vi "Set Exposure Time.vi"(8 "error in (no error)":errorcluster, 10 "Exposure Time (s)":dbl, 11 "Abstract Camera in":refnum<class "Abstract Camera.lvclass">) -> (0 "error out":errorcluster, 2 "Exposure Time (s) out":dbl, 3 "Abstract Camera out":refnum<class "Abstract Camera.lvclass">)   [LabVIEW 2019, in "Abstract Camera.lvclass"]
uses:
  Abstract Camera.lvclass
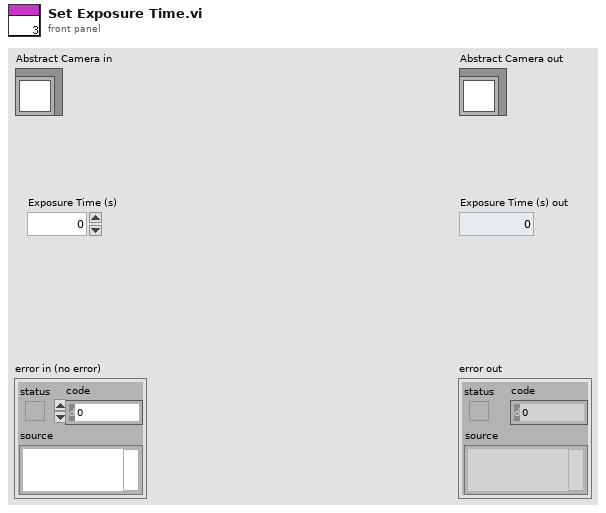
[diagram p1: front panel]
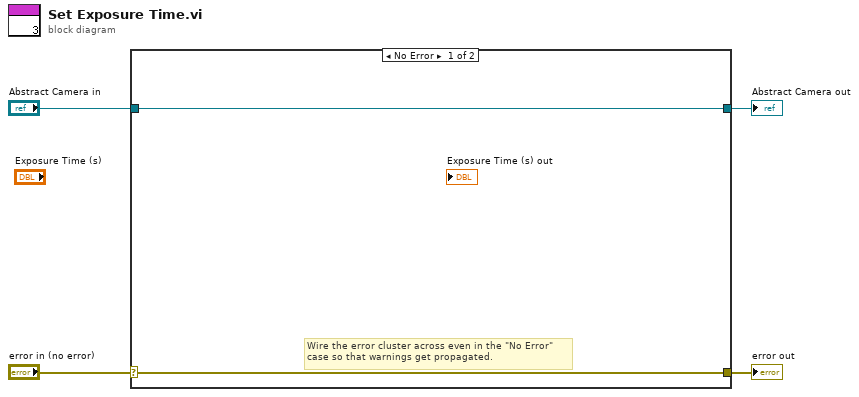
[diagram p0: block diagram]
diagram:
  n1 = case shown="No Error" "error in (no error)" {
    selector: "error in (no error)" -> [w5 w8]
    tunnel: [w5 w8] -> w3
    tunnel: [w6 w7] -> w1
    tunnel: "Abstract Camera in" -> [w6 w7]
    frame No Error {
      # "Wire the error cluster across even in the \"No Error\"\ncase so that warnings get propagated."
    }
    frame Error {
    }
  }
  "error out" <- w3
  "Abstract Camera out" <- w1
